vi "Motion_Error Handler.vi"(8 "error in (no error)":errorcluster, 10 "Exception Code":u8, 11 "TCP Connection Refnum in":refnum<k5>) -> (0 "error out":errorcluster, 3 "TCP Connection Refnum (dup)":refnum<k5>)   [LabVIEW 2010]
uses:
  <vilib>/NI Modbus.llb/MB Ethernet Master Query Read Discrete Inputs (poly).vi
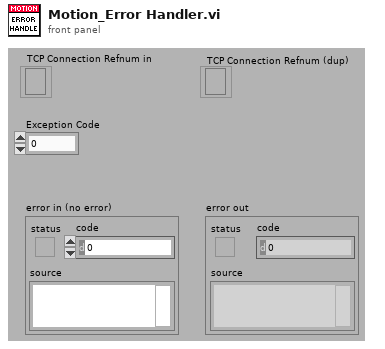
[diagram p1: front panel]
types:
  T1 = cluster{"[0]":bool, "[1]":bool, "[2]":bool, "[3]":bool, "[4]":bool}
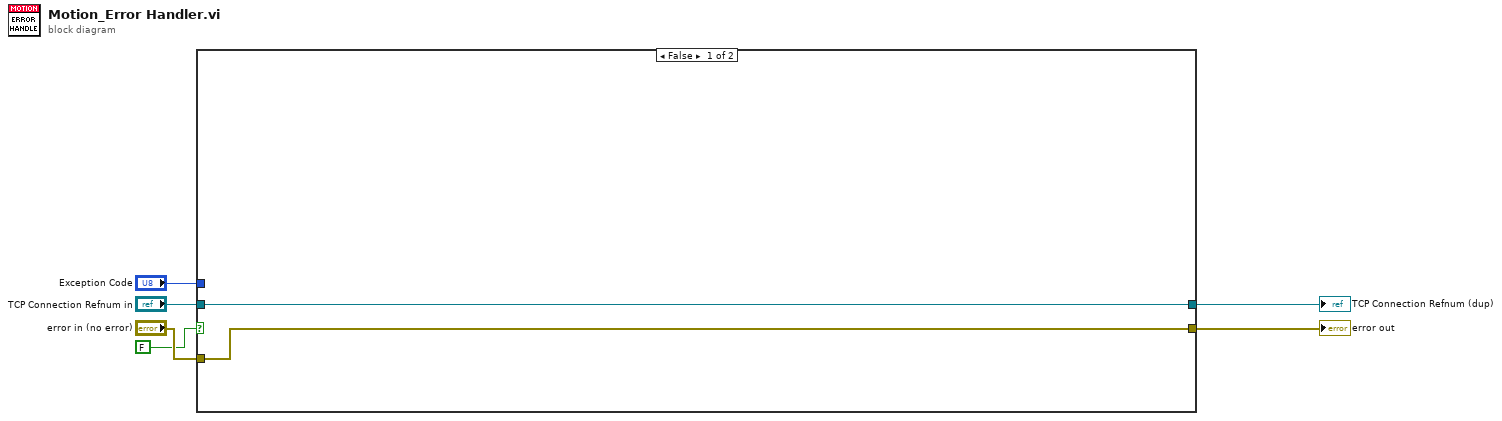
[diagram p0: block diagram]
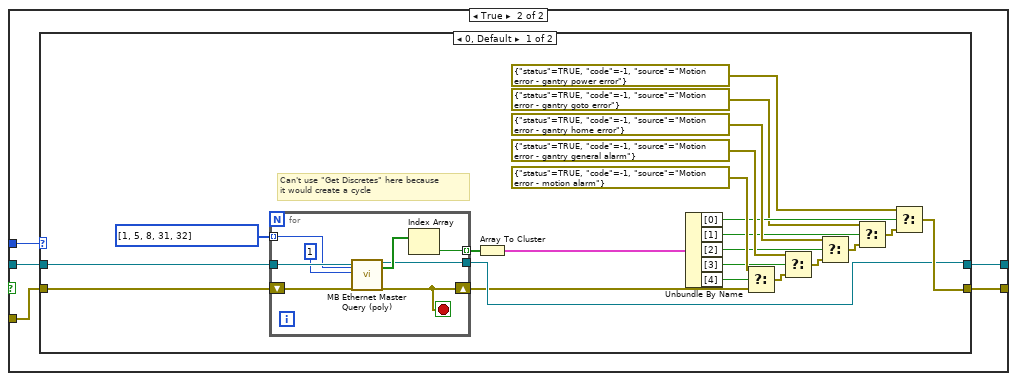
[diagram p2: hidden frame]
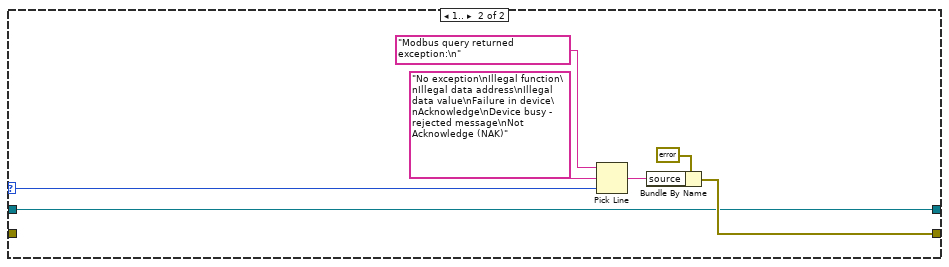
[diagram p3: hidden frame]
diagram:
  n1 = case shown="False" FALSE {
    tunnel: "Exception Code" -> [_ w13]
    tunnel: [w7 w12] -> w5
    tunnel: "TCP Connection Refnum in" -> [w8 w11]
    tunnel: [w8 w10] -> w3
    tunnel: "error in (no error)" -> [w7 w9]
    frame False {
    }
    frame True {
      n2 = case shown="0, Default" w13 {
        selector: w13 -> [_ w48]
        tunnel: [w21 w45] -> w12
        tunnel: w9 -> [w20 _]
        tunnel: w11 -> [w19 w44]
        tunnel: [w17 w44] -> w10
        frame 0, Default {
          # "Can't use \"Get Discretes\" here because\nit would create a cycle"
          n3 = for {
            tunnel: w19 -> [w42]
            tunnel: u16[] [1, 5, 8, 31, 32] -> [w41] mode=indexing
            tunnel: [w38] -> w17
            tunnel: [w37] -> w16 mode=indexing
            shift-right: [w36] -> w14
            shift-left: w20 -> [w43]
            stop <- w36 stop-if-true
            n4 = call-poly <vilib>:"MB Ethernet Master Query (poly).vi"("TCP Connection Refnum in"=w42, "Starting Address"=w41, "Quantity"=u16 1, "error in"=w43) -> ("TCP Connection Refnum (dup)"=w38:refnum<k5>, "Discrete Inputs"=w39:bool[], "error out"=w36:errorcluster)  [unwired: 12 in, 1 out]
            n5 = Index Array(array=w39) -> (element=w37:bool)  [unwired: 1 in]
          }
          n6 = Array To Cluster(array=w16) -> (cluster=w15:T1)
          n7 = Unbundle By Name(w15) -> ("[0]"=w24:bool, "[1]"=w25:bool, "[2]"=w29:bool, "[3]"=w32:bool, "[4]"=w35:bool)
          n8 = Select(t=errorcluster {"status"=TRUE, "code"=-1, "source"="Motion error - motion alarm"} ("error in (no error)"), s=w35, f=w14) -> (s? t:f=w33:errorcluster)
          n9 = Select(t=errorcluster {"status"=TRUE, "code"=-1, "source"="Motion error - gantry general alarm"} ("error in (no error)"), s=w32, f=w33) -> (s? t:f=w30:errorcluster)
          n10 = Select(t=errorcluster {"status"=TRUE, "code"=-1, "source"="Motion error - gantry home error"} ("error in (no error)"), s=w29, f=w30) -> (s? t:f=w27:errorcluster)
          n11 = Select(t=errorcluster {"status"=TRUE, "code"=-1, "source"="Motion error - gantry goto error"} ("error in (no error)"), s=w25, f=w27) -> (s? t:f=w26:errorcluster)
          n12 = Select(t=errorcluster {"status"=TRUE, "code"=-1, "source"="Motion error - gantry power error"} ("error in (no error)"), s=w24, f=w26) -> (s? t:f=w21:errorcluster)
        }
        frame 1.. {
          n13 = Pick Line(string ("")="Modbus query returned exception:\n", multi-line string="No exception\nIllegal function\nIllegal data address\nIllegal data value\nFailure in device\nAcknowledge\nDevice busy - rejected message\nNot Acknowledge (NAK)", line index=w48) -> (output string=w47:string)
          n14 = Bundle By Name(cluster=errorcluster {"status"=TRUE, "code"=-1, "source"=""} ("error IO"), "source"=w47) -> (w45:errorcluster)
        }
      }
    }
  }
  "error out" <- w5
  "TCP Connection Refnum (dup)" <- w3
